vi "Masking.vi"(8 "error in":errorcluster, 11 "Male/Female":T1=enum."Male") -> (0 "error out":errorcluster, 3 "Detected Frequency (Hz)":dbl format="%.2p")   [LabVIEW 2018, in "CollectionSupport.lvlib"]
uses:
  CollectionSupport.lvlib
  Controls/Male_Female.ctl
  Controls/MaskStates.ctl
  <vilib>/DAQmx/read.llb/DAQmx Read (Analog 1D Wfm NChan NSamp).vi
  <vilib>/DAQmx/create/channels.llb/DAQmx Create Channel (AI-Voltage-Basic).vi
  <vilib>/DAQmx/miscellaneous.llb/DAQmx Fill In Error Info.vi
  <vilib>/measure/matone.llb/Extract Single Tone Information 1 Chan.vi
  <vilib>/measure/NI_MAPro.lvlib
panel:
  out "task out":refnum<k21>
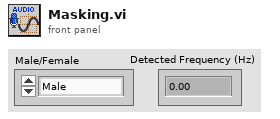
[diagram p1: front panel]
types:
  T1 = typedef "CollectionSupport.lvlib/Male_Female.ctl" = enum16{"Female", "Male"}
  T2 = typedef "CollectionSupport.lvlib/MaskStates.ctl" = enum16{"Start", "Connect", "Output", "Check", "Quit"}
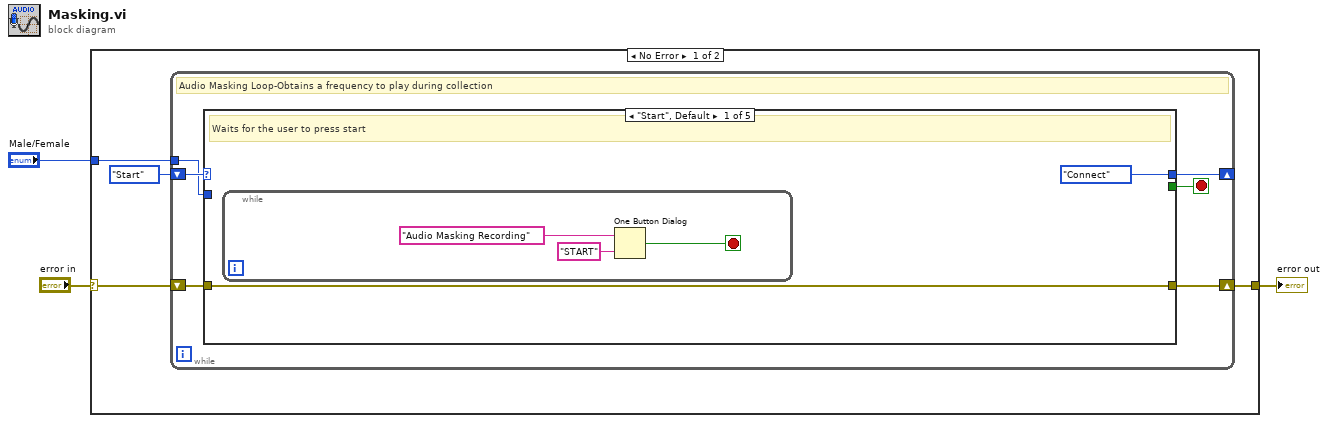
[diagram p0: block diagram]
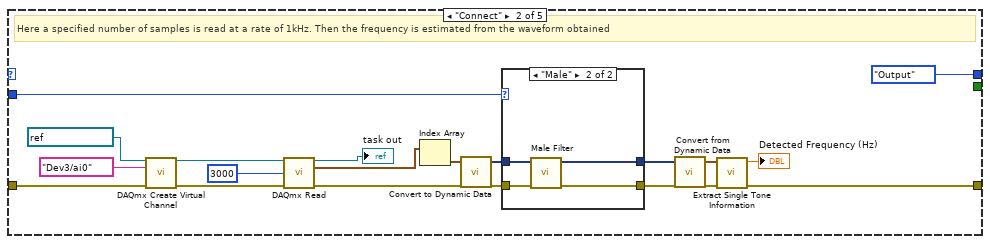
[diagram p2: hidden frame]
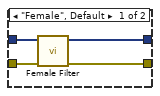
[diagram p3: hidden frame]
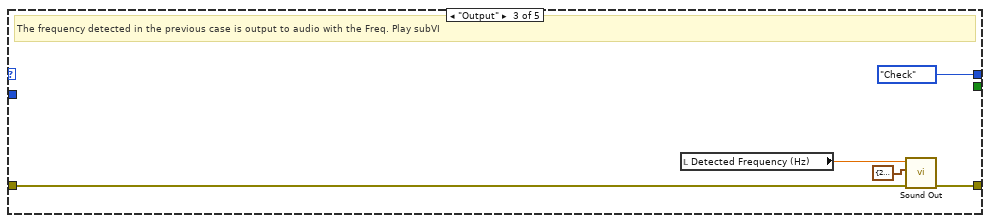
[diagram p4: hidden frame]
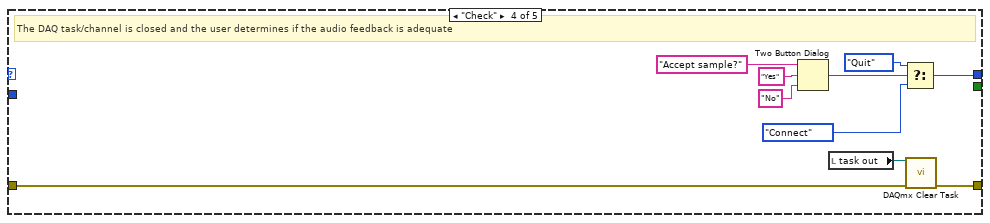
[diagram p5: hidden frame]
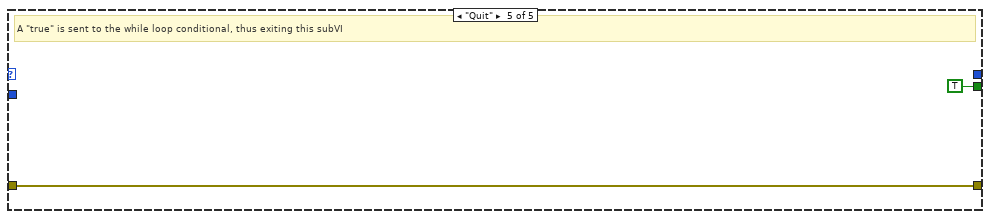
[diagram p6: hidden frame]
diagram:
  n1 = case shown="No Error" "error in" {
    selector: "error in" -> [w6 w62]
    tunnel: [w5 w62] -> w3
    tunnel: "Male/Female" -> [w4 _]
    frame No Error {
      n2 = while {
        shift-right: [w12] -> _
        shift-left: MaskStates."Start" ("First Case") -> [w13]
        shift-right: [w11] -> w5
        shift-left: w6 -> [w9]
        tunnel: w4 -> [w8]
        stop <- w10 stop-if-true
        # "Audio Masking Loop-Obtains a frequency to play during collection"
        n3 = case shown="\"Start\", Default" w13 {
          tunnel: [MaskStates."Connect" ("First Case") MaskStates."Output" ("First Case") MaskStates."Check" ("First Case") w55 _] -> w12
          tunnel: [w15 w23 w48 w53 w60] -> w11
          tunnel: [_ _ _ _ TRUE] -> w10
          tunnel: w9 -> [w15 w27 w49 w54 w60]
          tunnel: w8 -> [_ w19 _ _ _]
          frame "Start", Default {
            # "Waits for the user to press start"
            n4 = while {
              stop <- w16 stop-if-true
              n5 = One Button Dialog(message="Audio Masking Recording", button name ("OK")="START") -> (true=w16:bool)
            }
          }
          frame "Connect" {
            # "Here a specified number of samples is read at a rate of 1kHz. Then the frequency is estimated from the waveform obtained"
            n6 = call-poly <vilib>:"DAQmx Create Virtual Channel.vi"("task in"=refnum<k21> "AudioVolts", "physical channels"=tag "Dev3/ai0", "error in"=w27) -> ("task out"=w25:refnum<k21>, "error out"=w26:errorcluster)  [unwired: 11 in]
            n7 = call-poly <vilib>:"DAQmx Read.vi"("task/channels in"=w25, "number of samples per channel"=3000, "error in"=w26) -> ("task out"=→"task out":refnum<k21>, "data"=w35:waveform(dbl)[], "error out"=w30:errorcluster)  [unwired: 10 in]
            n8 = Index Array(array=w35) -> (element=w34:waveform(dbl))  [unwired: 1 in]
            n9 = call "Convert to Dynamic Data"("Waveform"=w34) -> ("Dynamic Data Type"=w33:dynamicdata)  [unwired: 3 in]
            n10 = case shown="\"Male\"" w19 {
              tunnel: w33 -> [w40 w44]
              tunnel: w30 -> [w39 w43]
              tunnel: [w38 w42] -> w21
              tunnel: [w37 w41] -> w20
              frame "Female", Default {
                n11 = call "Female Filter"("error in (no error)"=w39, "Signal"=w40) -> ("error out"=w38:errorcluster, "Filtered Signal"=w37:dynamicdata)  [unwired: 8 in]
              }
              frame "Male" {
                n12 = call "Male Filter"("error in (no error)"=w43, "Signal"=w44) -> ("error out"=w42:errorcluster, "Filtered Signal"=w41:dynamicdata)  [unwired: 8 in]
              }
            }
            n13 = call "Convert from Dynamic Data"("Dynamic Data Type"=w20) -> ("Waveform"=w32:waveform(dbl))  [unwired: 3 in]
            n14 = call-poly <vilib>:"Extract Single Tone Information.vi"("error in (no error)"=w21, "time signal in"=w32) -> ("error out"=w23:errorcluster, "detected frequency"=→"Detected Frequency (Hz)":dbl)  [unwired: 4 in, 4 out]
          }
          frame "Output" {
            # "The frequency detected in the previous case is output to audio with the Freq. Play subVI"
            n15 = local read "Detected Frequency (Hz)"() -> (w47:dbl)
            n16 = call "Sound Out.vi"("error in (no error)"=w49, "sampling info"=cluster{"Fs":dbl, "#s":dbl} {"Fs"=22050.0, "#s"=66150.0}, "Detected Frequency (Hz)"=w47) -> ("error out"=w48:errorcluster)  [unwired: 7 in, 1 out]
          }
          frame "Check" {
            # "The DAQ task/channel is closed and the user determines if the audio feedback is adequate"
            n17 = Two Button Dialog(message="Accept sample?", 1:"No" ("F button name (\"Cancel\")"), 2:"Yes" ("T button name (\"OK\")")) -> (T button?=w56:bool)
            n18 = local read "task out"() -> (w52:refnum<k21>)
            n19 = Select(t=MaskStates."Quit" ("First Case"), s=w56, f=MaskStates."Connect" ("First Case")) -> (s? t:f=w55:T2)
            n20 = call <vilib>:"DAQmx Clear Task.vi"("task in"=w52, "error in"=w54) -> ("error out"=w53:errorcluster)  [unwired: 13 in]
          }
          frame "Quit" {
            # "A \"true\" is sent to the while loop conditional, thus exiting this subVI"
          }
        }
      }
    }
    frame Error {
    }
  }
  "error out" <- w3
